vi "SCMP -Move AISAS.vi"(4 "FITS Header in":T3={"Wavelength (nm)"=530.15, "Exposure (s)"=0.05, "Tuning Delay (ms)"=1000.0, "Beam Type (-1/1)"=1.0, "Tuning Voltages"=[1.111, 2.222, 3.333, 4.444], "Observer"="observer", "Light Shapping Diffuser"=enum."In Beam", "Comment"="", "Data Type"=9, "Mod Cycles"=0, "SCD Calibration Optics"=enum."1 - Polarizer @0, I+Q", "SCD Emission Line Filter"=enum."1-557.6nm", "Cookbook"="", "COMP-S Calibration Wheel"=enum."Dark", "COMP-S Andover Filter Wheel"=enum."530.3nm/HWB 0.34nm (Fe XIV)", "FOV Rotation (deg)"=66.0, "Objective Lens Position (mm)"=0.0, "Occulter size"=0.0, "Time End"=timestamp(3382374145.421875 s since 1904-01-01), "Acc Exposure (s)"=0.0, "Time Stamp Array"=[], "Camera Serial Number"=[], "Camera Temp"=[], "Camera PI (mm)"=[], "Time Start"=timestamp(3382374145.421875 s since 1904-01-01), "Peripherals"={"ILX controler"=FALSE, "Zone temperatures"=FALSE, "Andor"=FALSE, "Andor 2"=FALSE, "PI Stages"=FALSE, "AISAS mechanisms"=FALSE, "AISAS Mech.lvclass"=refnum, "Zone temp ref"=variant, "FWs"=FALSE}, "FITS paths"=[], "Cameras"=enum."Andor", "load preset cbk"=FALSE, "periodic check count"=0} {"Camera PI (mm)" format="%_3g"; "Acc Exposure (s)" format="%^.3g"; "Occulter size" format="%.2f"; "Objective Lens Position (mm)" min=70.0 max=152.0 format="%.2f"; "FOV Rotation (deg)" format="%.1f"; "Data Type" items=["LIVE", "DARK", "FLAT", "CALI", "OBSE", "ABSO", "AURE", "TARG", "OBJE", "HOLE", "OREX", "THRO", "CHIP"]; "Exposure (s)" format="%^.3g"; "Wavelength (nm)" format="%_6g"}, 6 "Motors":bool=TRUE, 7 "Diffuser in":T2=enum."In Beam", 8 "error in (no error)":errorcluster, 9 "value changed arr":bool[](array[boolean]), 10 "Rotation in":dbl, 11 "Focus in":T1=70.0 min=70.0 max=152.0 format="%.2f") -> (0 "error out":errorcluster, 2 "New Rotation":dbl, 3 "New Focus":T1=70.0 min=70.0 max=152.0 format="%.2f", 5 "New Diffuser":T2=enum."In Beam")   [LabVIEW 2014]
uses:
  AISAS/Controls/Diffuser.ctl
  Controls/SCD - FITS Cluster.ctl
  AISAS/Mech/AISAS Mech.lvclass
  Controls/SCD - Calibration Optics Filter Wheel.ctl
  Controls/SCD - EDT - Emission Line Filter Wheel.ctl
  Controls/CoMP-S Controls/Polarization Optics Filter Wheel.ctl
  Controls/CoMP-S Controls/Emission Line Filter Wheel.ctl
  AISAS/Controls/focus.ctl
  Controls/peripherals.ctl
  Controls/Cameras select.ctl
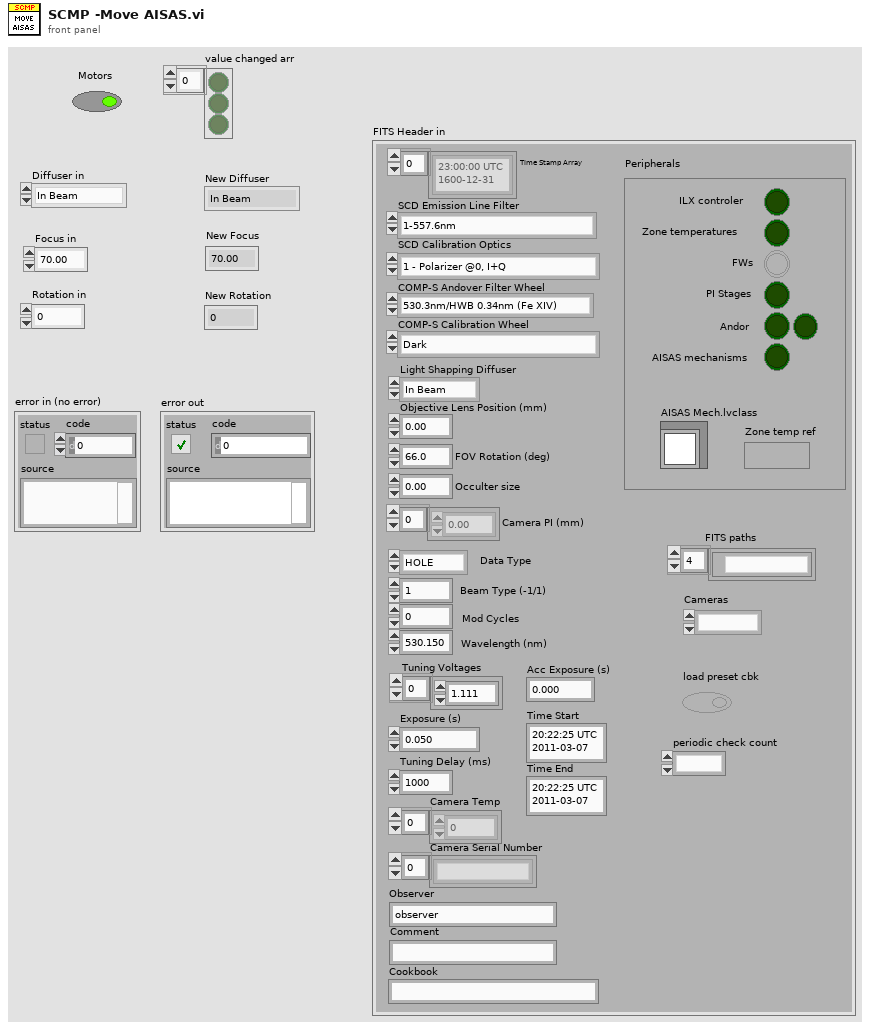
[diagram p1: front panel]
types:
  T1 = typedef "focus.ctl" = dbl
  T2 = typedef "Diffuser.ctl" = enum16{"Out of Beam", "In Beam"}
  T3 = typedef "SCD - FITS Cluster.ctl" = cluster{"Wavelength (nm)":dbl, "Exposure (s)":dbl, "Tuning Delay (ms)":dbl, "Beam Type (-1/1)":dbl, "Tuning Voltages":dbl[], "Observer":string, "Light Shapping Diffuser":T2, "Comment":string, "Data Type":u16, "Mod Cycles":u16, "SCD Calibration Optics":T4, "SCD Emission Line Filter":T5, "Cookbook":string, "COMP-S Calibration Wheel":T6, "COMP-S Andover Filter Wheel":T7, "FOV Rotation (deg)":dbl, "Objective Lens Position (mm)":T1, "Occulter size":dbl, "Time End":timestamp, "Acc Exposure (s)":dbl, "Time Stamp Array":timestamp[], "Camera Serial Number":string[], "Camera Temp":dbl[], "Camera PI (mm)":dbl[], "Time Start":timestamp, "Peripherals":T8, "FITS paths":path[], "Cameras":T9, "load preset cbk":bool, "periodic check count":i32}
  T4 = typedef "SCD - Calibration Optics Filter Wheel.ctl" = enum16{"1 - Polarizer @0, I+Q", "2 - Polarizer @90, I-Q", "3 - Polarizer @45, I+U", "4 - Polarizer @135, I-U", "5 - Polarizer @0, Retarder @45, I+V", "6 - Polarizer @0, Retarder @135, I-V", "7 - Dark", "8 - Clear", "9 - N/A"}
  T5 = typedef "SCD - EDT - Emission Line Filter Wheel.ctl" = enum16{"1-557.6nm", "2-587.6nm", "3-589.6nm", "4-630.2nm", "5-656.4nm", "6-849.8nm", "7-854.2nm", "8-866.2nm", "9-1083.0nm"}
  T6 = typedef "Polarization Optics Filter Wheel.ctl" = enum16{"Dark", "Clear", "Exchange Lens", "Polarizer @0, I+Q", "Polarizer @90, I-Q", "Polarizer @45, I+U", "Polarizer @135, I-U", "Polarizer @0, Retarder @45, I+V", "Polarizer @0, Retarder @135, I-V"}
  T7 = typedef "Emission Line Filter Wheel.ctl" = enum16{"530.3nm/HWB 0.34nm (Fe XIV)", "587.6nm/HBW 0.44nm (He I D3)", "637.5nm/HBW 0.53nm (Fe X)", "656.3nm/HBW 0.57nm (H-Alpha)", "789.2nm/HBW 0.85nm (Fe XI)", "854.2nm/HBW 1.01nm (Ca I)", "1074.7nm/HBW 2.34nm (Fe XIII)", "1079.8nm/HBW 1.64nm (Fe XIII)", "1083.0nm/HBW 1.66nm (He I)"}
  T8 = typedef "peripherals.ctl" = cluster{"ILX controler":bool, "Zone temperatures":bool, "Andor":bool, "Andor 2":bool, "PI Stages":bool, "AISAS mechanisms":bool, "AISAS Mech.lvclass":refnum<class "AISAS Mech.lvclass">, "Zone temp ref":variant, "FWs":bool}
  T9 = typedef "Cameras select.ctl" = enum16{"Andor", "GDR"}
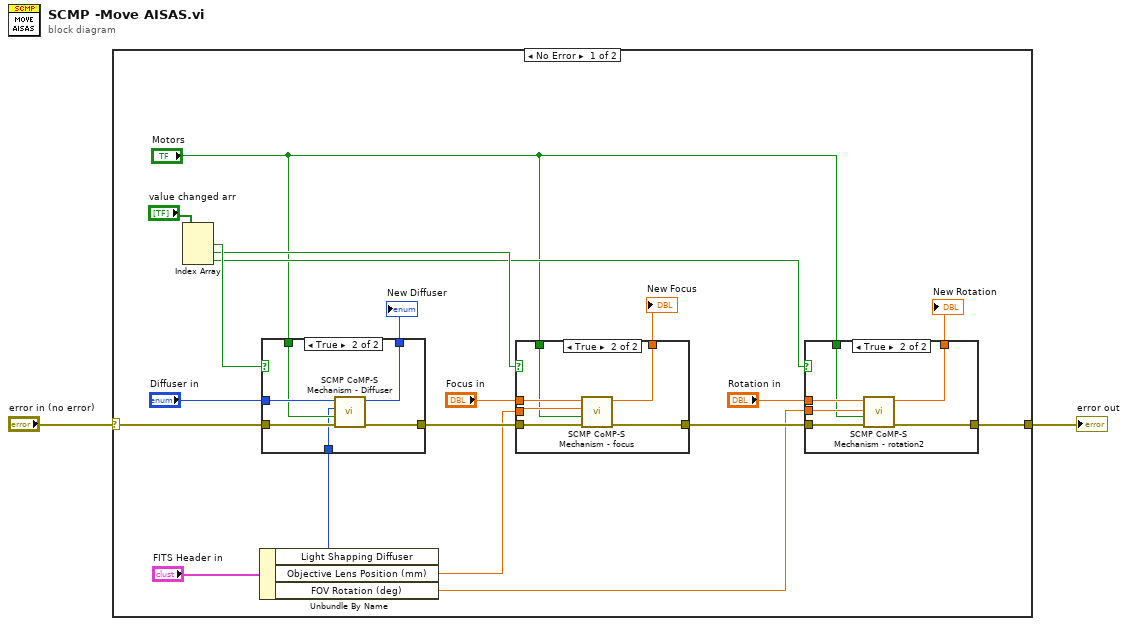
[diagram p0: block diagram]
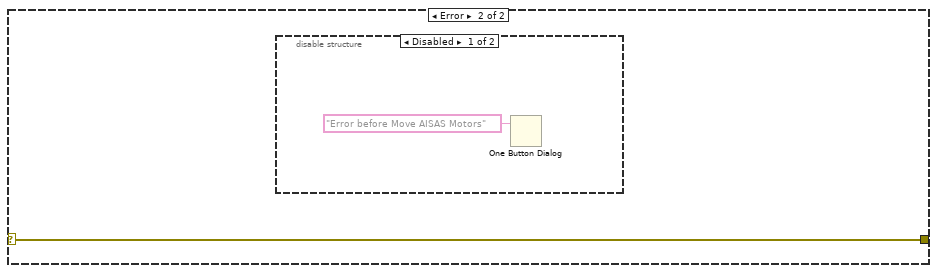
[diagram p5: hidden frame]
diagram:
  n1 = case shown="No Error" "error in (no error)" {
    selector: "error in (no error)" -> [w20 w46]
    tunnel: [w14 w46] -> w1
    frame No Error {
      n2 = Index Array(array="value changed arr") -> (element #1=w18:bool, element #2=w10:bool, element #3=w9:bool)  [unwired: 3 in]
      n3 = Unbundle By Name("FITS Header in") -> ("Light Shapping Diffuser"=w5:T2, "Objective Lens Position (mm)"=w12:T1, "FOV Rotation (deg)"=w11:dbl)
      n4 = case shown="True" w18 {
        tunnel: "Diffuser in" -> [w38 w45]
        tunnel: w20 -> [w39 w44]
        tunnel: [w39 w42] -> w17
        tunnel: "Motors" -> [_ w43]
        tunnel: [w38 w41] -> w7
        tunnel: w5 -> [_ w40]
        frame False {
        }
        frame True {
          n5 = call "SCMP CoMP-S Mechanism - Diffuser.vi"("error in (no error)"=w44, "Auto Motors"=w43, "Old Diffuser"=w40, "Desired Diffuser"=w45) -> ("error out"=w42:errorcluster, "New Diffuser"=w41:T2)  [unwired: 6 in]
        }
      }
      "New Diffuser" <- w7
      n6 = case shown="True" w10 {
        tunnel: "Focus in" -> [w30 w35]
        tunnel: w17 -> [w31 w36]
        tunnel: [w31 w37] -> w15
        tunnel: w12 -> [_ w34]
        tunnel: "Motors" -> [_ w33]
        tunnel: [w30 w32] -> w3
        frame False {
        }
        frame True {
          n7 = call "SCMP CoMP-S Mechanism - focus.vi"("error in (no error)"=w36, "Auto Motors"=w33, "Old Focus"=w34, "Desired Focus"=w35) -> ("error out"=w37:errorcluster, "Focus out"=w32:dbl)  [unwired: 6 in]
        }
      }
      "New Focus" <- w3
      n8 = case shown="True" w9 {
        tunnel: "Rotation in" -> [w22 w29]
        tunnel: w15 -> [w23 w28]
        tunnel: [w23 w27] -> w14
        tunnel: w11 -> [_ w26]
        tunnel: "Motors" -> [_ w25]
        tunnel: [w22 w24] -> w6
        frame False {
        }
        frame True {
          n9 = call "SCMP CoMP-S Mechanism - rotation2.vi"("error in (no error)"=w28, "Auto Motors"=w25, "Old Rotation"=w26, "Desired Rotation"=w29) -> ("error out"=w27:errorcluster, "Rotation out"=w24:dbl)  [unwired: 6 in]
        }
      }
      "New Rotation" <- w6
    }
    frame Error {
      n10 = disable-structure shown="Disabled" {
        frame Disabled {
          n11 = One Button Dialog(message="Error before Move AISAS Motors") -> ()  [unwired: 1 in, 1 out]
        }
        frame Enabled {
        }
      }
    }
  }
  "error out" <- w1
